vi "Wave generator 2.vi"() -> ()   [LabVIEW 2023]
uses:
  <vilib>/Analysis/2dsp.llb/Real FFT.vi
  <vilib>/express/express analysis/Spectral/Block/exnSpectralBlock spectral measurements peak poly.vi
  <vilib>/express/express analysis/Spectral/Block/exnSpectralBlock spectral measurements peak DDT.vi
  <vilib>/express/express analysis/Spectral/XNode/ExpressSpectralMeasurementsBlockNode.xnode
  <vilib>/Analysis/NI_AALPro.lvlib
panel:
  out "max value":dbl
  out "NXT Style graph 2":dbl[](graph)
  out "Normalised Frequency":dbl
  in  "Amplitude":dbl=1.0
  in  "Frequency":dbl=10.0
  out "?":dbl[](graph)
  out "NXT Style graph":dbl[][](graph)
  in  "FFT Size":i32
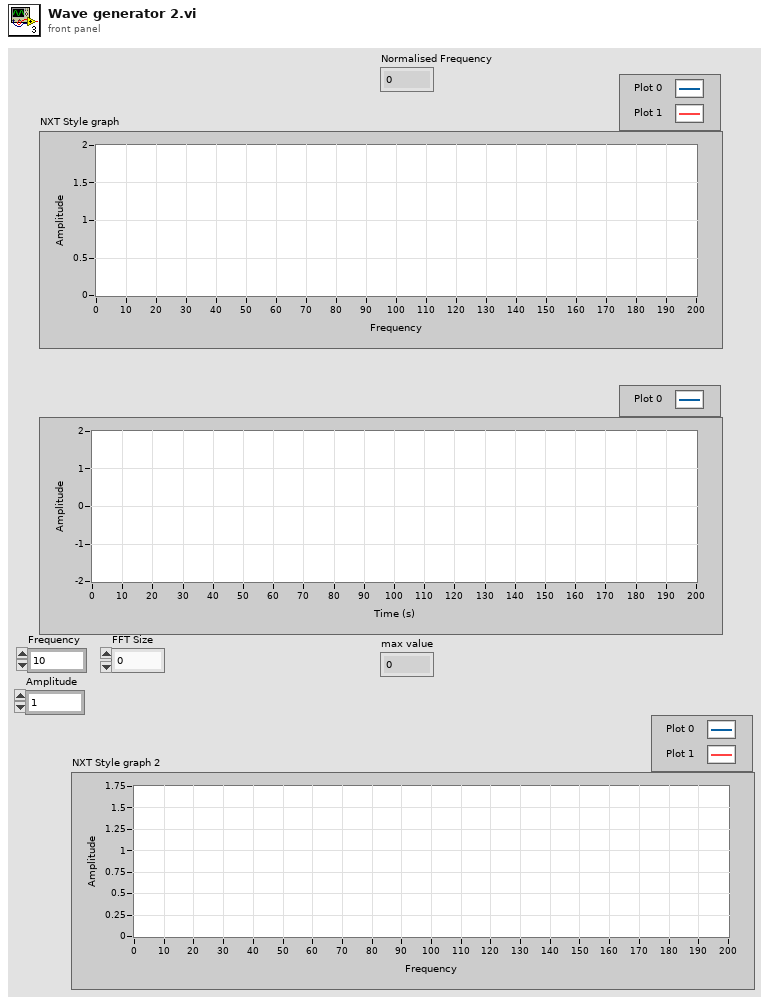
[diagram p1: front panel]
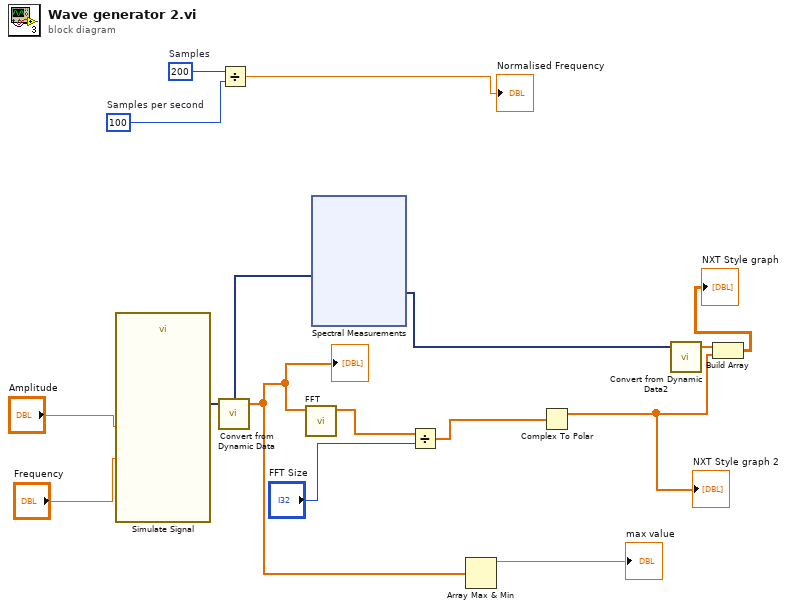
[diagram p0: block diagram]
diagram:
  w3 = 100  # Samples per second
  w4 = 200  # Samples
  n1 = call "Simulate Signal"("Frequency"="Frequency", "Amplitude"="Amplitude") -> ("Sine"=w12:dynamicdata)  [unwired: 12 in, 1 out]
  n2 = call "Convert from Dynamic Data"("Dynamic Data Type"=w12) -> ("Array"=w2:dbl[])  [unwired: 3 in]
  "?" <- w2
  n3 = Divide(x=w4, y=w3) -> (x/y=→"Normalised Frequency":dbl)
  n4 = call-poly <vilib>:"FFT.vi"("X"=w2) -> ("FFT {X}"=w15:cdb[])  [unwired: 9 in, 1 out]
  n5 = xnode "Spectral Measurements"("Signals"=w12) -> ("FFT - (Peak)"=w11:dynamicdata)  [unwired: 1 in, 2 out]
  n6 = Divide(x=w15, y="FFT Size") -> (x/y=w13:cdb[])
  n7 = Array Max & Min(array=w2) -> (max value=→"max value":dbl)  [unwired: 3 out]
  n8 = Complex To Polar(r * e^(i*theta)=w13) -> (r=w5:dbl[])  [unwired: 1 out]
  "NXT Style graph 2" <- w5
  n9 = call "Convert from Dynamic Data2"("Dynamic Data Type"=w11) -> ("Array"=w10:dbl[])  [unwired: 3 in]
  n10 = Build Array(w10, w5) -> (→"NXT Style graph":dbl[][])
